vi "Get Black Box File Data.vi"(2 "Delete File?":bool, 3 "Inst Name":string, 4 "Black Box Filename":path=path "C:/Cambustion/User Interface/Black Box/Black Box - ESN 251 - Channel 1.txt") -> (0 "Channel Values":string[](array[string]), 1 "Channel Names":string[](array[string]))   [LabVIEW 2022 SP3]
uses:
  <vilib>/Analysis/baseanly.llb/Mean (DBL).vi
  Globals/Meas_global.vi
  <vilib>/Analysis/NI_AALBase.lvlib
panel:
  in  "Numeric":i32=35
  out "Output":dbl[](graph)
  out "Head Temp":dbl[](graph)
  in  "History length":i32=1500
  out "All channels":string[](array[string])
  out "Flame Temp":dbl[](graph)
  out "resulting string":string
  out "Channel":string
  out "ESN":string
  out "array":string[][](array[string])
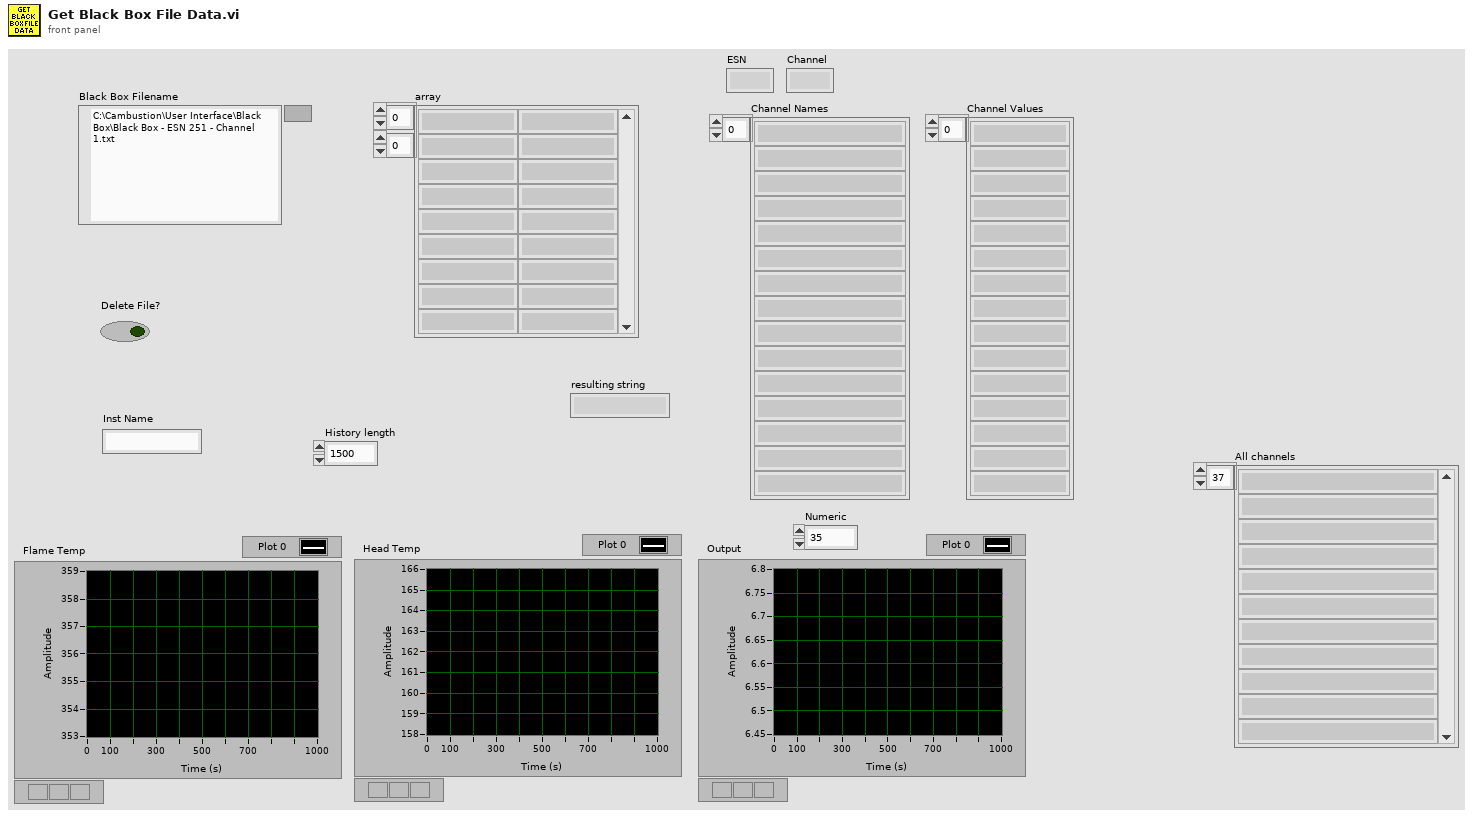
[diagram p1: front panel]
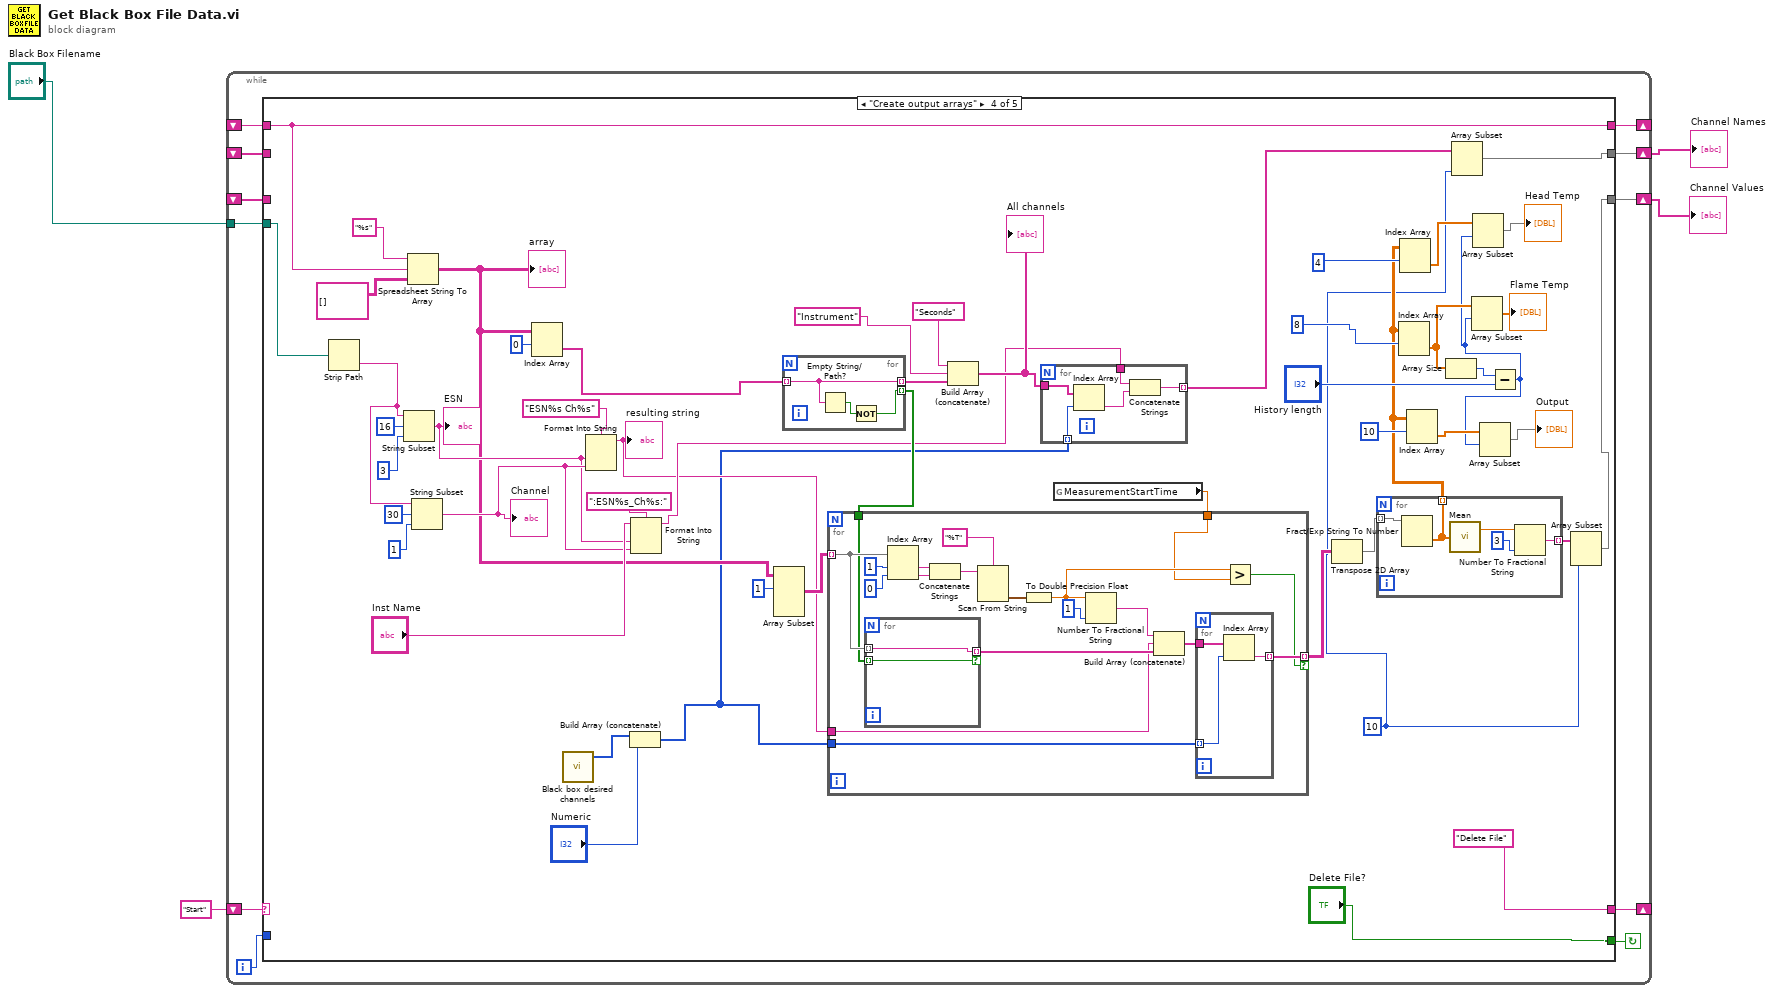
[diagram p0: block diagram]
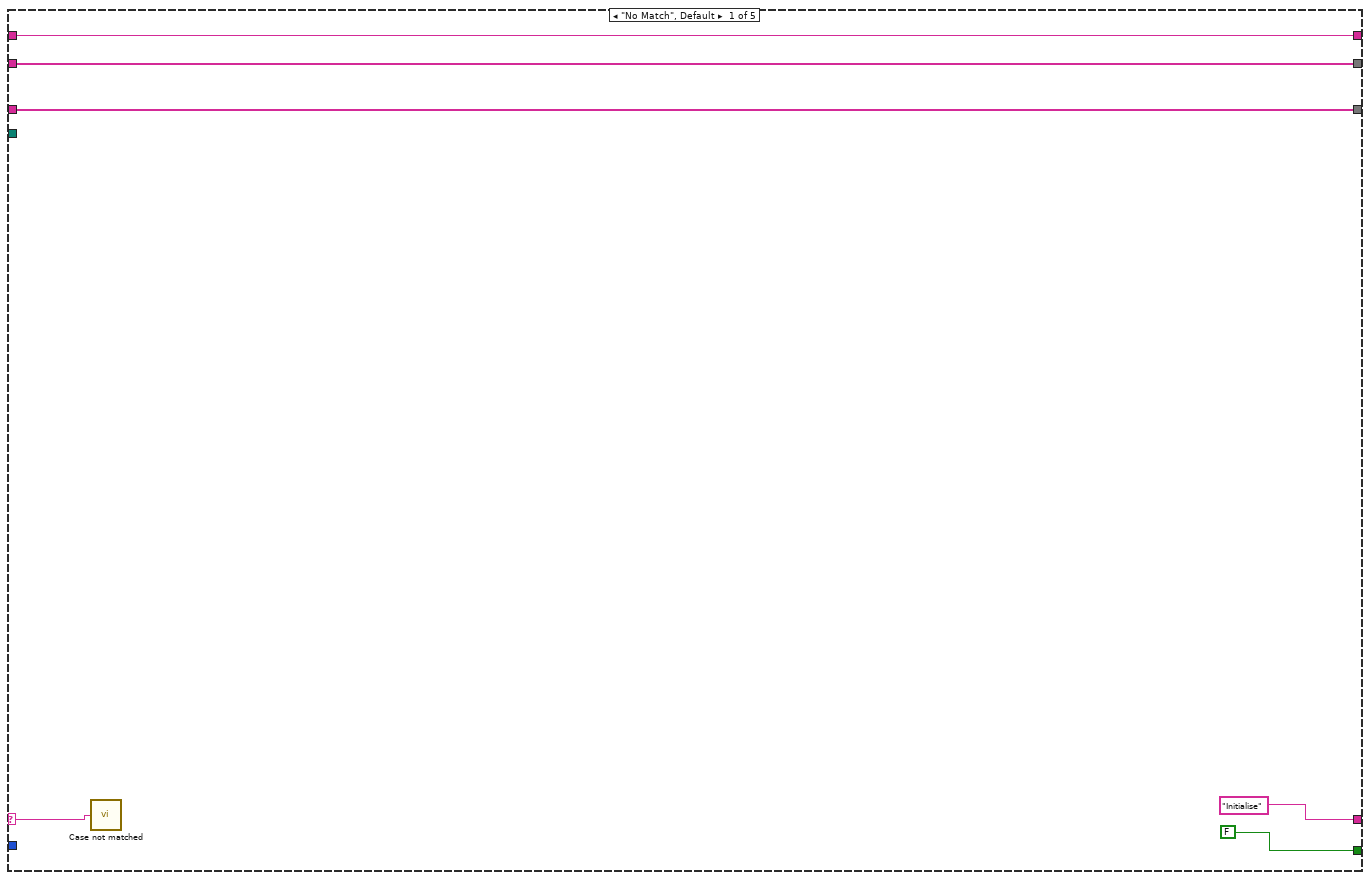
[diagram p2: hidden frame]
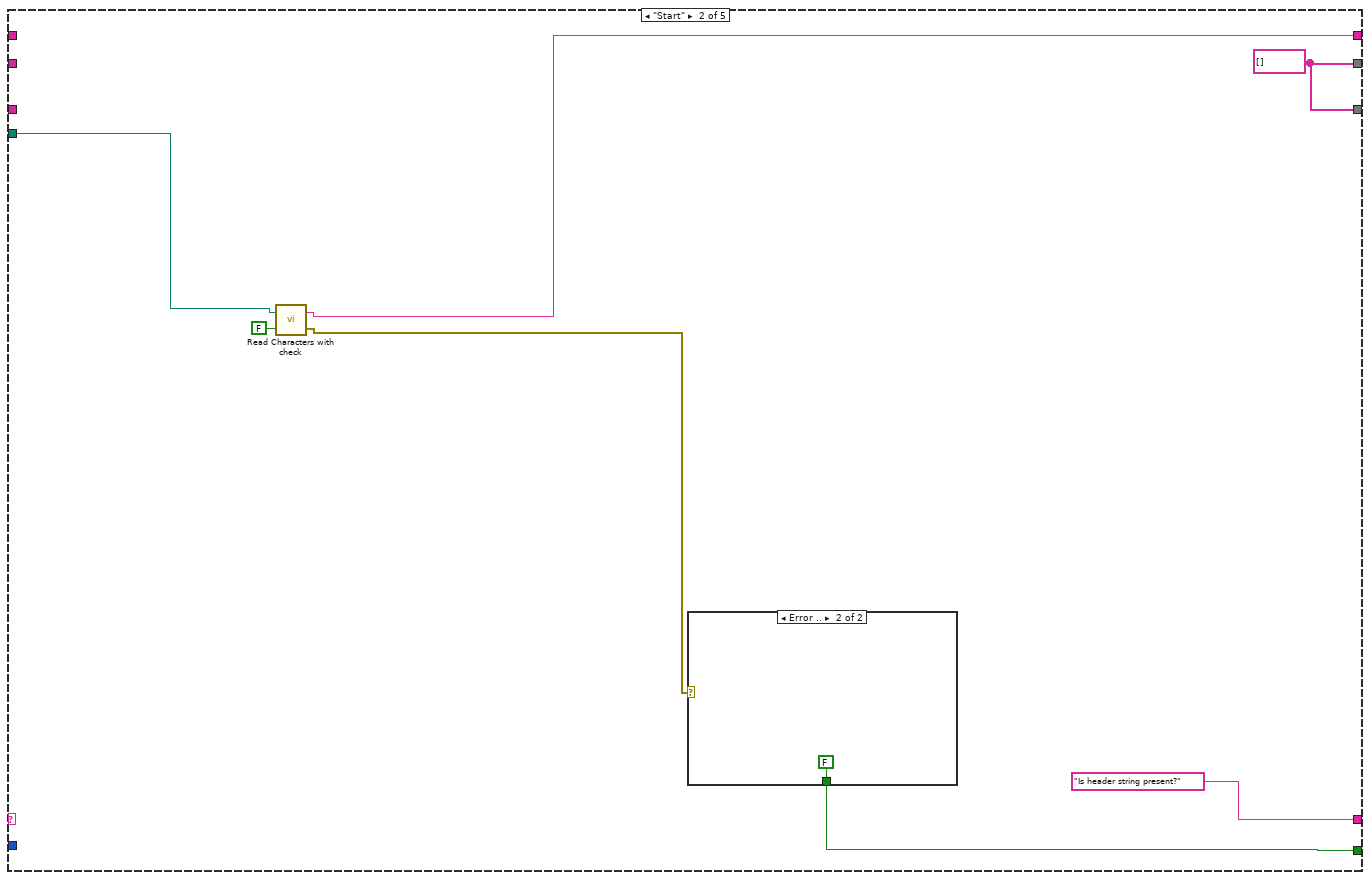
[diagram p3: hidden frame]
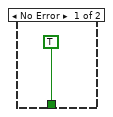
[diagram p4: hidden frame]
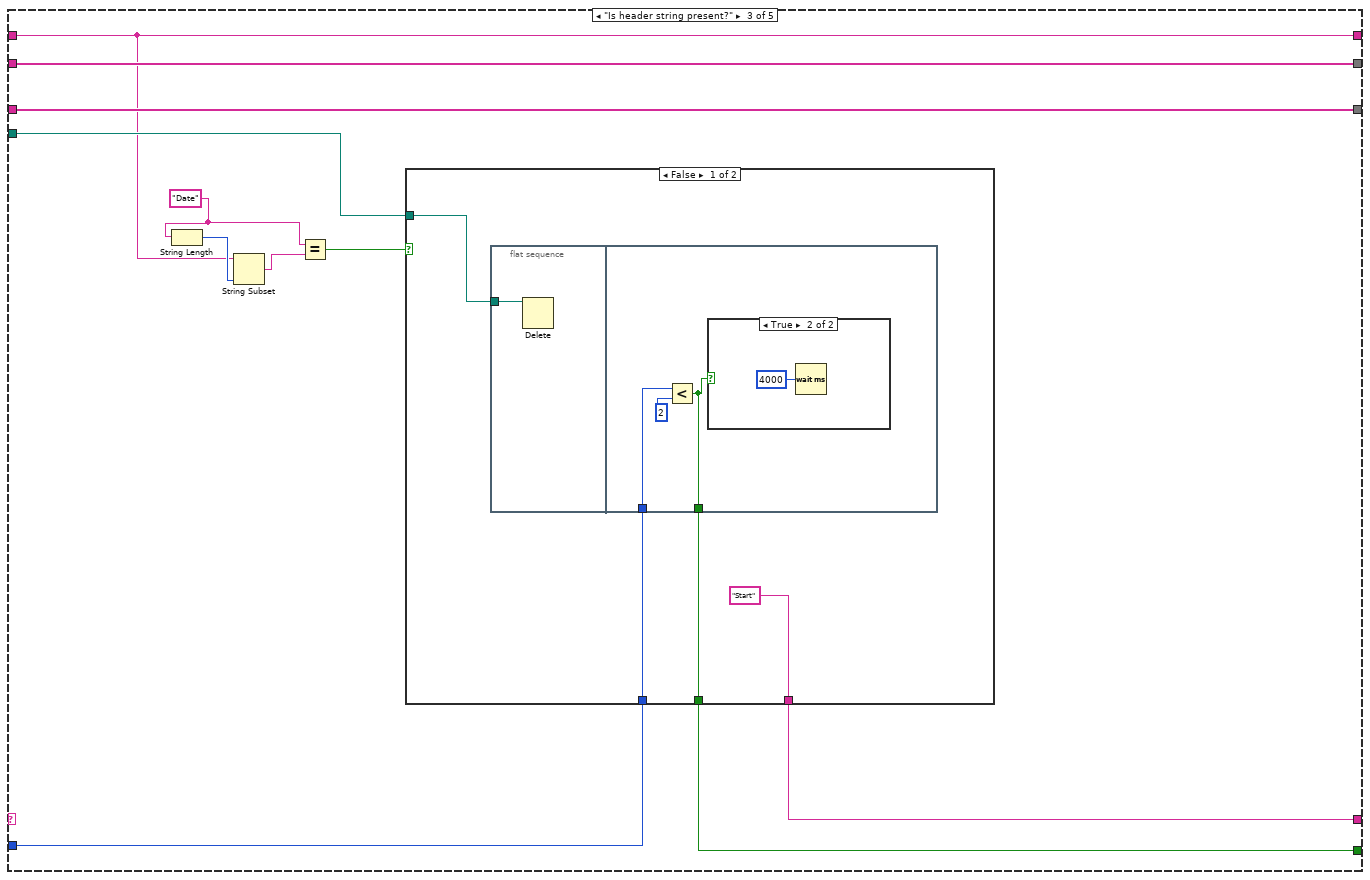
[diagram p5: hidden frame]
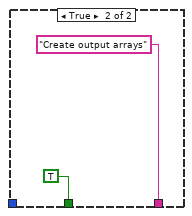
[diagram p7: hidden frame]
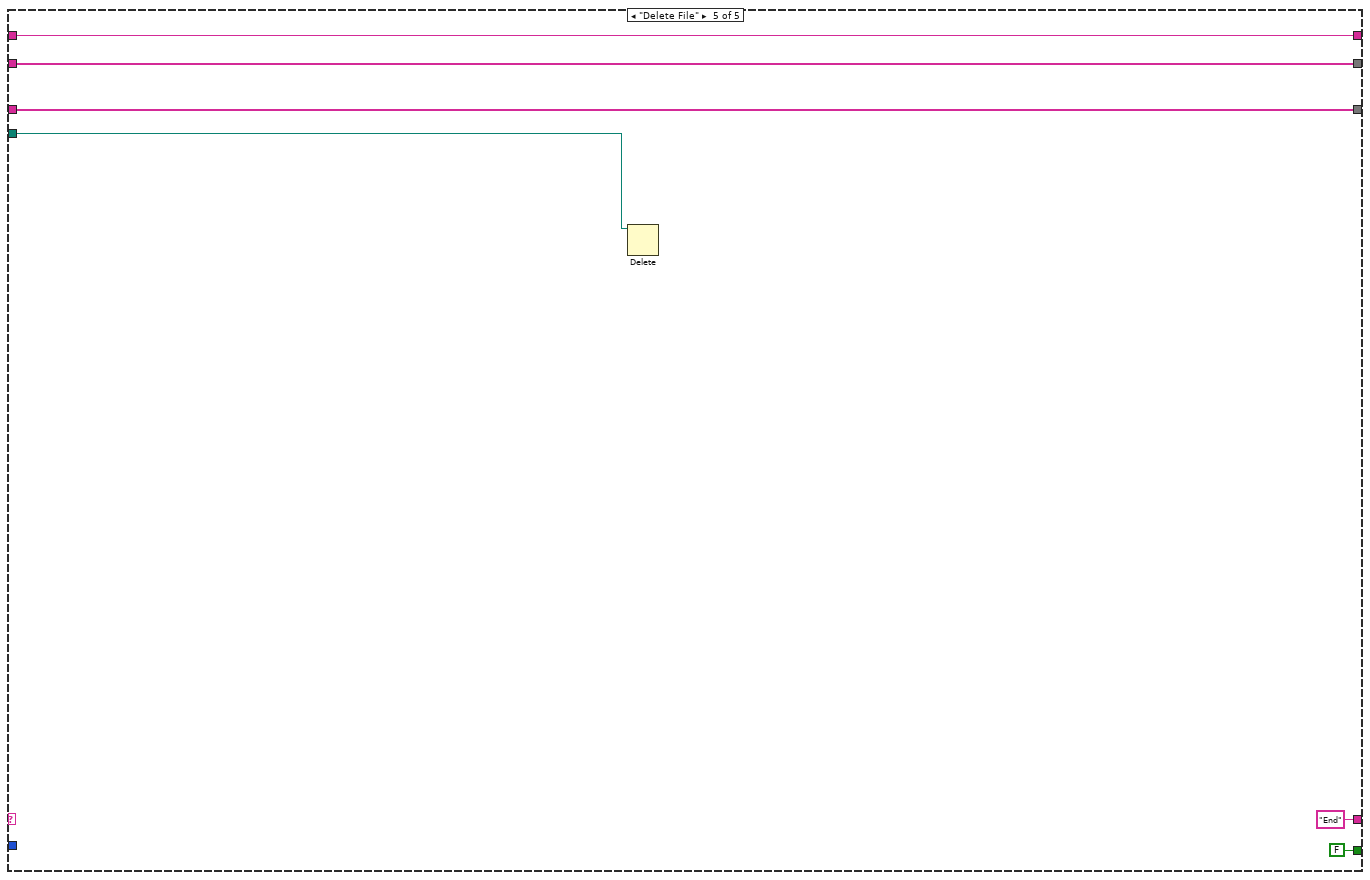
[diagram p8: hidden frame]
diagram:
  n1 = while {
    shift-left: "Start" -> [w13]
    shift-right: [w14] -> _
    shift-right: [w12] -> w2
    shift-left: _ -> [w10]
    shift-right: [w11] -> w3
    shift-left: _ -> [w9]
    shift-right: [w7] -> _
    shift-left: _ -> [w6]
    tunnel: "Black Box Filename" -> [w8]
    i -> [w5]
    stop <- w15 continue-if-true
    n2 = case shown="\"Create output arrays\"" w13 {
      selector: w13 -> [w19 _ _ _ _]
      tunnel: [FALSE w27 w33 "Delete File?" FALSE ("Delete File?")] -> w15
      tunnel: ["Initialise" "Is header string present?" w35 "Delete File" "End"] -> w14
      tunnel: [w17 w26 w41 w59 w144] -> w12
      tunnel: [w16 w26 w40 w57 w145] -> w11
      tunnel: w10 -> [w17 _ w41 _ w144]
      tunnel: w9 -> [w16 _ w40 _ w145]
      tunnel: w8 -> [_ w25 w34 w77 w146]
      tunnel: [w18 w24 w31 w76 w143] -> w7
      tunnel: w6 -> [w18 _ w31 w76 w143]
      tunnel: w5 -> [_ _ w32 _ _]
      frame "No Match", Default {
        n3 = call "Case not matched.vi"("Case Name not Matched"=w19) -> ()
      }
      frame "Start" {
        w26 = string[] [] ("Channel Values")
        n4 = call "Read Characters with check.vi"("Call EnFlo Error Handler?"=FALSE, "file (use dialog)"=w25) -> ("error out"=w23:errorcluster, "Read String"=w24:string)
        n5 = case shown="Error .." w23 {
          tunnel: [TRUE FALSE] -> w27
          frame No Error {
          }
          frame Error {
          }
        }
      }
      frame "Is header string present?" {
        w37 = "Date"
        n6 = String Length(string=w37) -> (length=w39:i32)
        n7 = String Subset(string=w31, length (rest)=w39) -> (substring=w38:string)  [unwired: 1 in]
        n8 = Equal?(x=w37, y=w38) -> (x = y?=w36:bool)
        n9 = case shown="False" w36 {
          tunnel: ["Start" "Create output arrays"] -> w35
          tunnel: w34 -> [w45 _]
          tunnel: [w42 TRUE] -> w33
          tunnel: w32 -> [w43 _]
          frame False {
            n10 = flat-sequence {
              tunnel: w45 -> [w46]
              tunnel: w43 -> [w49]
              tunnel: [w47] -> w42
              frame #0 {
                n11 = Delete(path (use dialog)=w46) -> ()  [unwired: 4 in, 3 out]
              }
              frame #1 {
                n12 = Less?(x=w49, y=2) -> (x < y?=w47:bool)
                n13 = case shown="True" w47 {
                  frame False {
                  }
                  frame True {
                    n14 = Wait (ms)(milliseconds to wait=u32 4000) -> ()  [unwired: 1 out]
                  }
                }
              }
            }
          }
          frame True {
          }
        }
      }
      frame "Create output arrays" {
        w56 = 10 ("length")
        n15 = Strip Path(path=w77) -> (name=w92:string)  [unwired: 1 out]
        n16 = String Subset(string=w92, offset (0)=16, length (rest)=3 ("length (rest)")) -> (substring=w94:string)
        "ESN" <- w94
        n17 = Spreadsheet String To Array(format string="%s", spreadsheet string=w76, array type (2D Dbl)=string[][] []) -> (array=w91:string[][])  [unwired: 1 in]
        "array" <- w91
        n18 = String Subset(string=w92, offset (0)=30, length (rest)=1 ("length (rest)")) -> (substring=w95:string)
        "Channel" <- w95
        n19 = Index Array(array=w91, index (row)=0) -> (element=w90:string[])  [unwired: 1 in]
        n20 = call "Black box desired channels.vi"() -> ("Indicies"=w55:i32[])  [unwired: 4 in, 1 out]
        n21 = Format Into String(format string="ESN%s Ch%s", w94, w95) -> (resulting string=w93:string)  [unwired: 2 in, 1 out]
        "resulting string" <- w93
        n22 = Build Array (concatenate)(w55, "Numeric") -> (w54:i32[])
        n23 = Format Into String(format string=":ESN%s_Ch%s:", initial string="Inst Name", w94, w95) -> (resulting string=w96:string)  [unwired: 1 in, 1 out]
        n24 = Array Subset(array=w91, index (row)=1 ("index")) -> (w97:string[][])  [unwired: 3 in]
        n25 = for {
          tunnel: [w116] -> w98 mode=indexing if=w115
          tunnel: w90 -> [w116] mode=indexing
          tunnel: [w115] -> w99 mode=indexing
          n26 = Empty String/Path?(string/path=w116) -> (empty?=w117:bool)
          n27 = Not(x=w117) -> (.not. x?=w115:bool)
        }
        n28 = Build Array (concatenate)("Seconds", "Instrument", w98) -> (w100:string[])
        "All channels" <- w100
        n29 = for {
          tunnel: w100 -> [w114]
          tunnel: w54 -> [w113] mode=indexing
          tunnel: w96 -> [w111]
          tunnel: [w110] -> w60 mode=indexing
          n30 = Index Array(array=w114, index=w113) -> (element=w112:string)
          n31 = Concatenate Strings(w111, w112) -> (w110:string)
        }
        n32 = global read "Meas_global.vi" "MeasurementStartTime"() -> (w74:dbl)
        n33 = for {
          tunnel: w97 -> [w130] mode=indexing
          tunnel: [w125] -> w101 mode=indexing if=w123
          tunnel: w99 -> [w129]
          tunnel: w93 -> [w128]
          tunnel: w54 -> [w126]
          tunnel: w74 -> [w118]
          n34 = for {
            tunnel: [w141] -> w131 mode=indexing if=w140
            tunnel: w130 -> [w141] mode=indexing
            tunnel: w129 -> [w140] mode=indexing
          }
          n35 = Index Array(array=w130, index #1=1 ("index"), index #2=0 ("index")) -> (element #1=w121:string, element #2=w136:string)
          n36 = Concatenate Strings(w121, w136) -> (w122:string)
          n37 = Scan From String(format string="%T", input string=w122) -> (output 1=w124:timestamp)  [unwired: 3 in, 3 out]
          n38 = To Double Precision Float(number=w124) -> (double precision float=w119:dbl)
          n39 = Number To Fractional String(number=w119, precision (6)=i16 1) -> (F-format string=w120:string)  [unwired: 2 in]
          n40 = Build Array (concatenate)(w120, w128, w131) -> (w127:string[])
          n41 = for {
            tunnel: w127 -> [w139]
            tunnel: w126 -> [w138] mode=indexing
            tunnel: [w137] -> w125 mode=indexing
            n42 = Index Array(array=w139, index=w138) -> (element=w137:string)
          }
          n43 = Greater?(x=w119, y=w118) -> (0:w123:bool)
        }
        n44 = Transpose 2D Array(2D array=w101) -> (transposed array=w102:string[][])
        n45 = for {
          tunnel: w102 -> [w109] mode=indexing
          tunnel: [w106] -> w58 mode=indexing
          tunnel: [w105] -> w64 mode=indexing
          n46 = Fract/Exp String To Number(string=w109) -> (number=w105:dbl[])  [unwired: 3 in, 1 out]
          n47 = call-poly <vilib>:"Mean.vi"("X"=w105) -> ("mean"=w108:dbl)  [unwired: 1 out]
          n48 = Number To Fractional String(number=w108, precision (6)=i16 3) -> (F-format string=w106:string)  [unwired: 2 in]
        }
        n49 = Index Array(array=w64, index (row)=8) -> (element=w71:dbl[])  [unwired: 1 in]
        n50 = Index Array(array=w64, index (row)=4) -> (element=w68:dbl[])  [unwired: 1 in]
        n51 = Index Array(array=w64, index (row)=10) -> (element=w63:dbl[])  [unwired: 1 in]
        n52 = Array Size(array=w71) -> (size(s)=w73:i32)
        n53 = Array Subset(array=w60, length=w56) -> (w59:string[])  [unwired: 1 in]
        n54 = Subtract(x=w73, y="History length") -> (x-y=w62:i32)
        n55 = Array Subset(array=w71, index=w62) -> (→"Flame Temp":dbl[])  [unwired: 1 in]
        n56 = Array Subset(array=w68, index=w62) -> (→"Head Temp":dbl[])  [unwired: 1 in]
        n57 = Array Subset(array=w63, index=w62) -> (→"Output":dbl[])  [unwired: 1 in]
        n58 = Array Subset(array=w58, length=w56) -> (w57:string[])  [unwired: 1 in]
      }
      frame "Delete File" {
        n59 = Delete(path (use dialog)=w146) -> ()  [unwired: 4 in, 3 out]
      }
    }
  }
  "Channel Values" <- w3
  "Channel Names" <- w2
